vi "Record Path.vi"(9 "Record Path":bool) -> ()   [LabVIEW 2020]
uses:
  Framework/Robot Global Data.vi
  <vilib>/Analysis/Matrix/Numeric/Conversions/Matrix To Array - RM.vi
  <vilib>/Utility/file.llb/Write Delimited Spreadsheet (DBL).vi
  <vilib>/Analysis/Matrix/NI_Matrix.lvlib
panel:
  out "path":path
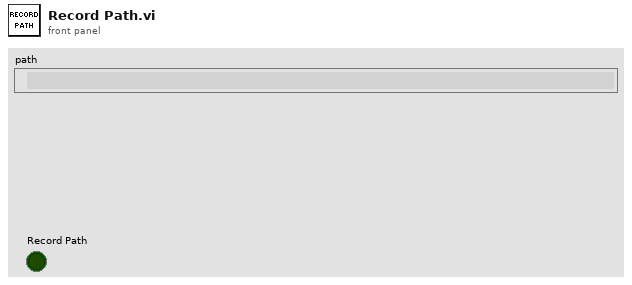
[diagram p1: front panel]
types:
  T1 = typedef "NI_Matrix.lvlib/RealMatrix.ctl" = dbl[][]
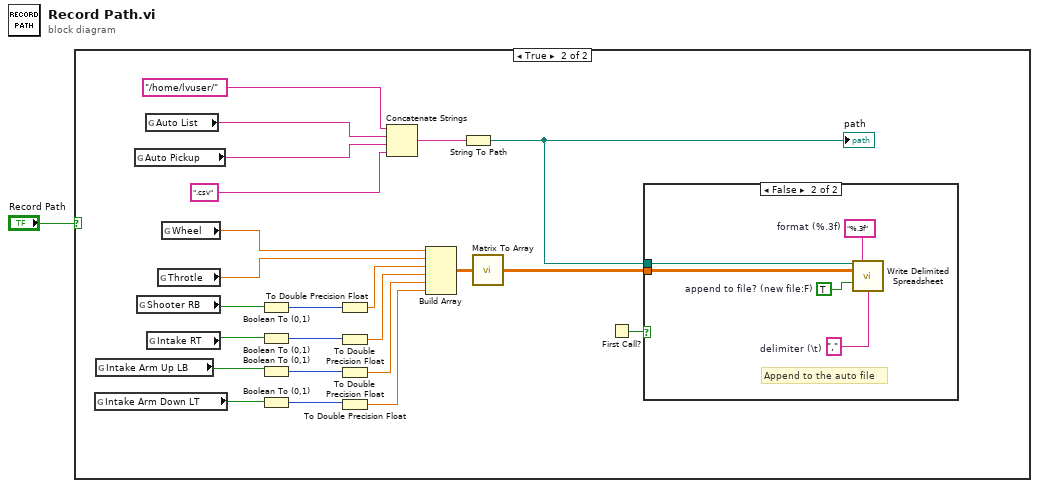
[diagram p0: block diagram]
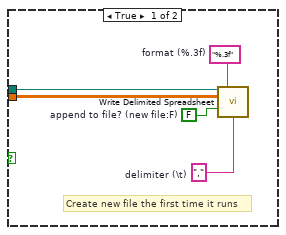
[diagram p3: hidden frame]
diagram:
  n1 = case shown="True" "Record Path" {
    frame False {
    }
    frame True {
      n2 = global read "Robot Global Data.vi" "Intake Arm Down LT"() -> (w6:bool)
      n3 = global read "Robot Global Data.vi" "Intake Arm Up LB"() -> (w7:bool)
      n4 = global read "Robot Global Data.vi" "Auto Pickup"() -> (w4:string)
      n5 = global read "Robot Global Data.vi" "Shooter RB"() -> (w9:bool)
      n6 = global read "Robot Global Data.vi" "Auto List"() -> (w5:string)
      n7 = global read "Robot Global Data.vi" "Intake RT"() -> (w8:bool)
      n8 = global read "Robot Global Data.vi" "Throtle"() -> (w10:dbl)
      n9 = global read "Robot Global Data.vi" "Wheel"() -> (w11:dbl)
      n10 = Boolean To (0,1)(Boolean=w9) -> (0, 1=w22:i16)
      n11 = Boolean To (0,1)(Boolean=w8) -> (0, 1=w21:i16)
      n12 = Boolean To (0,1)(Boolean=w7) -> (0, 1=w20:i16)
      n13 = Boolean To (0,1)(Boolean=w6) -> (0, 1=w19:i16)
      n14 = To Double Precision Float(number=w22) -> (double precision float=w18:dbl)
      n15 = To Double Precision Float(number=w21) -> (double precision float=w17:dbl)
      n16 = To Double Precision Float(number=w20) -> (double precision float=w16:dbl)
      n17 = To Double Precision Float(number=w19) -> (double precision float=w15:dbl)
      n18 = Concatenate Strings("/home/lvuser/", w5, w4, ".csv") -> (w12:string)
      n19 = Build Array(w11, w10, w18, w17, w16, w15) -> (w24:T1)
      n20 = String To Path(string=w12) -> (path=w3:path)
      "path" <- w3
      n21 = call-poly <vilib>:"Matrix To Array.vi"("Real Matrix"=w24) -> ("Real 2D Array"=w23:dbl[][])
      n22 = First Call?() -> (First Call?: T/F=w2:bool)
      n23 = case shown="False" w2 {
        tunnel: w23 -> [w29 w34]
        tunnel: w3 -> [w25 w30]
        frame True {
          w27 = FALSE  # append to file? (new file:F)
          w28 = "%.3f"  # format (%.3f)
          w26 = ","  # delimiter (\t)
          # "Create new file the first time it runs"
          n24 = call-poly <vilib>:"Write Delimited Spreadsheet.vi"("file path (dialog if empty)"=w25, "format (%.3f)"=w28, "2D data"=w29, "append to file? (new file:F)"=w27, "delimiter (\\t)"=w26) -> ()  [unwired: 9 in, 2 out]
        }
        frame False {
          w32 = TRUE  # append to file? (new file:F)
          w33 = "%.3f"  # format (%.3f)
          w31 = ","  # delimiter (\t)
          # "Append to the auto file"
          n25 = call-poly <vilib>:"Write Delimited Spreadsheet.vi"("file path (dialog if empty)"=w30, "format (%.3f)"=w33, "2D data"=w34, "append to file? (new file:F)"=w32, "delimiter (\\t)"=w31) -> ()  [unwired: 9 in, 2 out]
        }
      }
    }
  }
